vi "Update TTL - Ronen.vi"(8 "error in (no error)":errorcluster, 9 "TTL.lvclass":refnum<class "TTL.lvclass">, 11 "Pressure Control in":refnum<class "Pressure Control.lvclass">) -> (0 "error out":errorcluster, 3 "Pressure Control out":refnum<class "Pressure Control.lvclass">)   [LabVIEW 2014, in "Pressure Control.lvclass"]
uses:
  Pressure Control.lvclass
  TTL/TTL.lvclass
  Pressure Control.lvclass/Pressure Control.ctl
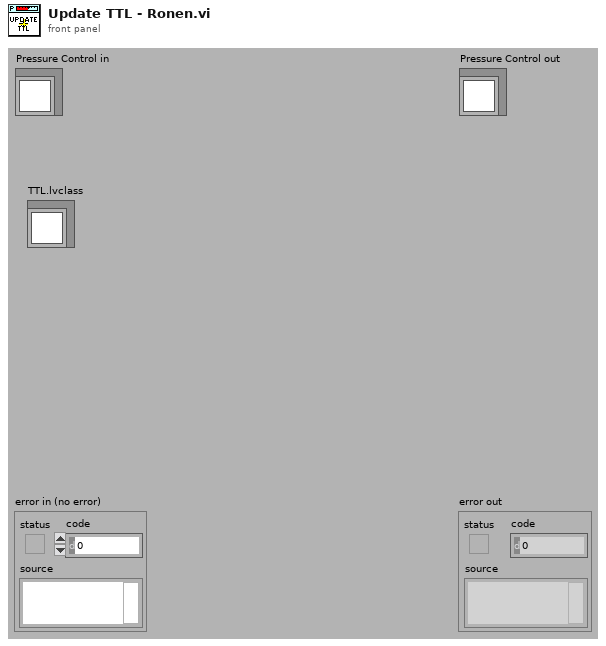
[diagram p1: front panel]
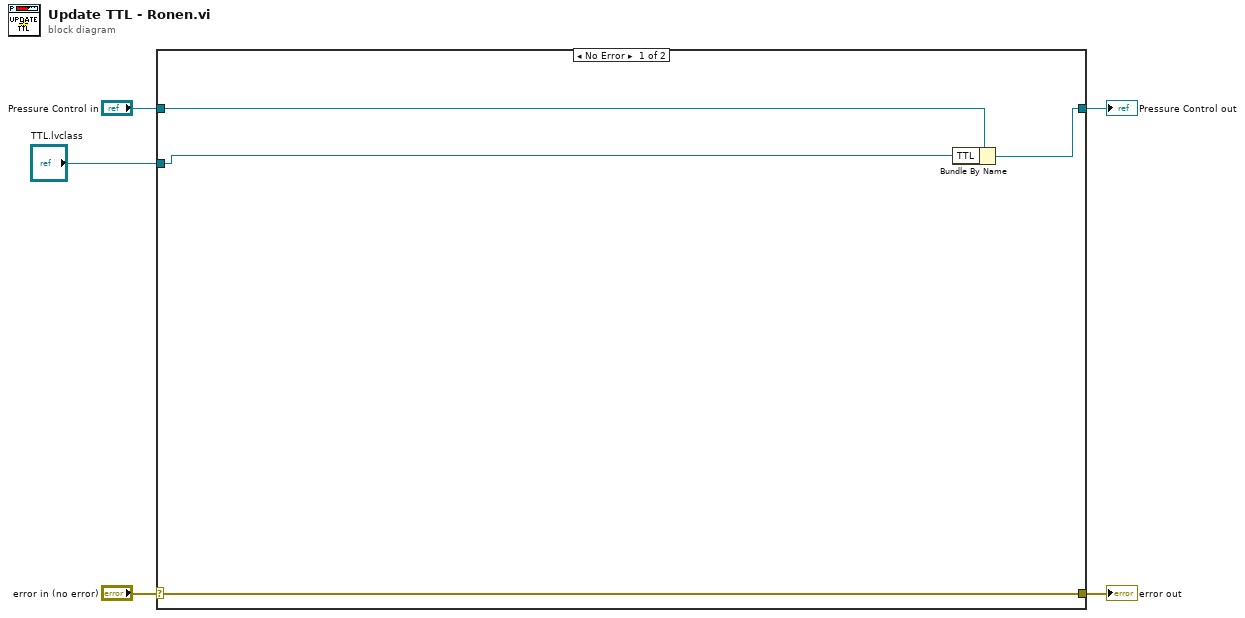
[diagram p0: block diagram]
diagram:
  n1 = case shown="No Error" "error in (no error)" {
    selector: "error in (no error)" -> [w9 w11]
    tunnel: [w9 w11] -> w4
    tunnel: [w7 w10] -> w2
    tunnel: "Pressure Control in" -> [w8 w10]
    tunnel: "TTL.lvclass" -> [w6 _]
    frame No Error {
      n2 = Bundle By Name(cluster=w8, "TTL"=w6) -> (w7:refnum<class "Pressure Control.lvclass">)
    }
    frame Error {
    }
  }
  "error out" <- w4
  "Pressure Control out" <- w2
